vi "Dual output square wave 180 out of phase.vi"(8 "error in (no error)":errorcluster, 11 "VISA resource name":refnum<visa-resource-name>="USB0::0x1AB1::0x0641::DG4E202501630::INSTR") -> (0 "error out":errorcluster)   [LabVIEW 2018]
uses:
  <instrlib>/RIGOL DG4000 Series/Public/Configure/Configure Standard Waveform(Square).vi
  <instrlib>/RIGOL DG4000 Series/Public/Configure/Configure Waveform Characteristics(Shape).vi
  <instrlib>/RIGOL DG4000 Series/Public/Configure/Configure Waveform Characteristics(Phase).vi
  <instrlib>/RIGOL DG4000 Series/RIGOL DG4000 Series.lvlib
panel:
  in  "Duty Cycle (50 %) 1":dbl=45.0
  in  "Duty Cycle (50 %) 2":dbl=45.0
  in  "Phase (0 Degree) 2":dbl
  in  "Phase (0 Degree) 1":dbl
  in  "DC Offset (0 V) 1":dbl=1.65
  in  "DC Offset (0 V) 2":dbl=1.65
  in  "Enable Align (F: Disable) 2":bool=TRUE
  in  "Enable Output 2":bool=TRUE
  in  "Enable Align (F: Disable) 1":bool=TRUE
  in  "Enable Output 1":bool=TRUE
  in  "Frequency 1":dbl
  in  "Frequency 2":dbl=180.0
  in  "Waveform Shape (0: Sinusoid) 2":i32(ring)=1 items=["Sinusoid", "Square", "Ramp", "Pulse", "Noise", "User", "Harmonic", "Custom", "DC", "AbsSine", "AbsSineHalf", "AmpALT", "AttALT", "GaussPulse", "NegRamp", "NPulse", "PPulse", "SineTra", "SineVer", "StairDn", "StairUD", "StairUp", "Trapezia", "BandLimited", "Butterworth", "Chebyshev1", "Chebyshev2", "Combin", "CPulse", "CWPulse", "DampedOsc", "DualTone", "Gamma", "GateVibr", "LEMPulse", "MCNoise", "Discharge", "Pahcur", "Quake", "Radar", "Ripple", "RoundHalf", "RoundPM", "StepResp", "SwingOsc", "TV", "Voice", "AM", "FM", "PM", "PWM", "PFM", "Cardiac", "EOG", "EEG", "EMG", "Pulseilogram", "ResSpeed", "LFPulse", "Tens1", "Tens2", "Tens3", "Lgnition", "ISO16750-2 SP", "ISO16750-2 VR", "ISO7637-2 TP1", "ISO7637-2 TP2A", "ISO7637-2 TP2B", "ISO7637-2 TP3A", "ISO7637-2 TP3B", "ISO7637-2 TP4", "ISO7637-2 TP5A", "ISO7637-2 TP5B", "SCR", "Surge", "Airy", "Besselj", "Bessely", "Cauchy", "Cubic", "Dirichlet", "Erf", "Erfc", "Erfclnv", "Erflnv", "ExpFall", "ExpRise", "Gauss", "HaverSine", "Laguerre", "Laplace", "Legend", "Log", "LogNormal", "Lorentz", "Maxwell", "Rayleigh", "Versiera", "Weibull", "ARB_X2", "CosH", "CosInt", "Cot", "CotHCon", "CotHPro", "CscCon", "CscPro", "CscHCon", "CscHPro", "RecipCon", "RecipPro", "SecCon", "SecPro", "SecH", "Sinc", "SinH", "SinInt", "Sqrt", "Tan", "TanH", "ACos", "ACosH", "ACotCon", "ACotPro", "ACotHCon", "ACotHPro", "ACscCon", "ACscPro", "ACscHCon", "ACscHPro", "ASecCon", "ASsePro", "ASecH", "ASin", "ASinH", "ATan", "ATanH", "Barlett", "BarthannWin", "Blackman", "BlackmanH", "BlackmanWin", "Boxcar", "ChebWin", "FlattopWin", "Hamming", "Hanning", "Kaiser", "NuttallWin", "ParzenWin", "TaylorWin", "Triang", "TukeyWin"]
  in  "Output Channel (1: Channel 1) 2":i32(ring)=2 items=["Channel 1"=1, "Channel 2"=2]
  in  "Amplitude (0.1 Vpp) 2":dbl=3.3
  in  "Amplitude (0.1 Vpp) 1":dbl=3.3
  in  "Output Channel (1: Channel 1)":i32(ring)=1 items=["Channel 1"=1, "Channel 2"=2]
  in  "Waveform Shape (0: Sinusoid) 1":i32(ring)=1 items=["Sinusoid", "Square", "Ramp", "Pulse", "Noise", "User", "Harmonic", "Custom", "DC", "AbsSine", "AbsSineHalf", "AmpALT", "AttALT", "GaussPulse", "NegRamp", "NPulse", "PPulse", "SineTra", "SineVer", "StairDn", "StairUD", "StairUp", "Trapezia", "BandLimited", "Butterworth", "Chebyshev1", "Chebyshev2", "Combin", "CPulse", "CWPulse", "DampedOsc", "DualTone", "Gamma", "GateVibr", "LEMPulse", "MCNoise", "Discharge", "Pahcur", "Quake", "Radar", "Ripple", "RoundHalf", "RoundPM", "StepResp", "SwingOsc", "TV", "Voice", "AM", "FM", "PM", "PWM", "PFM", "Cardiac", "EOG", "EEG", "EMG", "Pulseilogram", "ResSpeed", "LFPulse", "Tens1", "Tens2", "Tens3", "Lgnition", "ISO16750-2 SP", "ISO16750-2 VR", "ISO7637-2 TP1", "ISO7637-2 TP2A", "ISO7637-2 TP2B", "ISO7637-2 TP3A", "ISO7637-2 TP3B", "ISO7637-2 TP4", "ISO7637-2 TP5A", "ISO7637-2 TP5B", "SCR", "Surge", "Airy", "Besselj", "Bessely", "Cauchy", "Cubic", "Dirichlet", "Erf", "Erfc", "Erfclnv", "Erflnv", "ExpFall", "ExpRise", "Gauss", "HaverSine", "Laguerre", "Laplace", "Legend", "Log", "LogNormal", "Lorentz", "Maxwell", "Rayleigh", "Versiera", "Weibull", "ARB_X2", "CosH", "CosInt", "Cot", "CotHCon", "CotHPro", "CscCon", "CscPro", "CscHCon", "CscHPro", "RecipCon", "RecipPro", "SecCon", "SecPro", "SecH", "Sinc", "SinH", "SinInt", "Sqrt", "Tan", "TanH", "ACos", "ACosH", "ACotCon", "ACotPro", "ACotHCon", "ACotHPro", "ACscCon", "ACscPro", "ACscHCon", "ACscHPro", "ASecCon", "ASsePro", "ASecH", "ASin", "ASinH", "ATan", "ATanH", "Barlett", "BarthannWin", "Blackman", "BlackmanH", "BlackmanWin", "Boxcar", "ChebWin", "FlattopWin", "Hamming", "Hanning", "Kaiser", "NuttallWin", "ParzenWin", "TaylorWin", "Triang", "TukeyWin"]
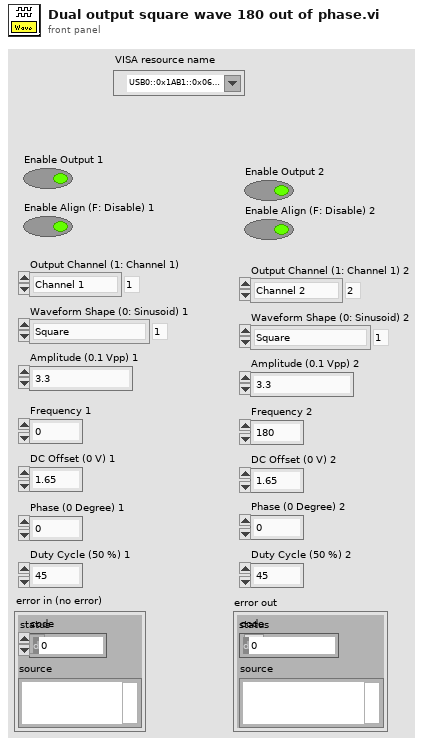
[diagram p1: front panel]
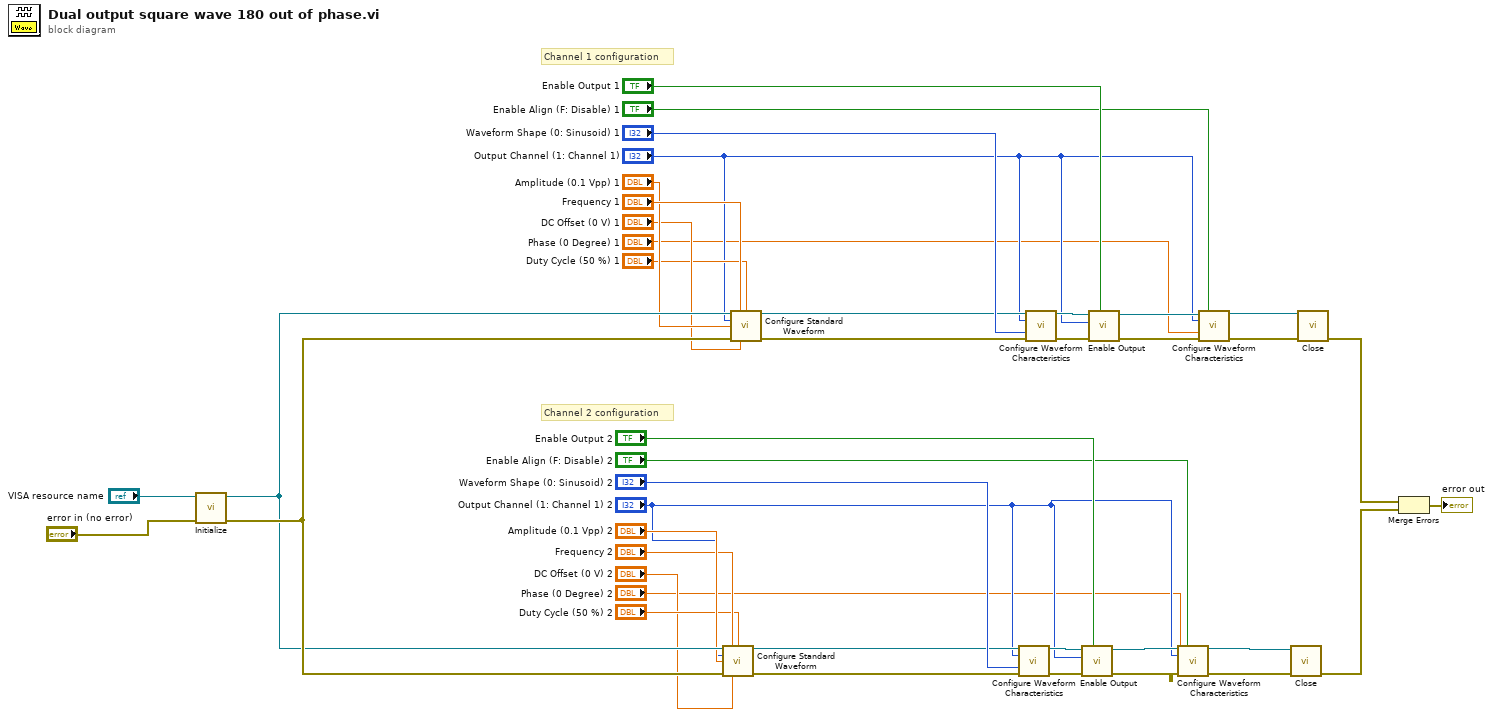
[diagram p0: block diagram]
diagram:
  # "Channel 2 configuration"
  # "Channel 1 configuration"
  n1 = call <instrlib>:"Initialize.vi"("error in (no error)"="error in (no error)", "VISA resource name"="VISA resource name") -> ("error out"=w34:errorcluster, "VISA resource name out"=w31:refnum<visa-resource-name>)  [unwired: 3 in, 5 out]
  n2 = call-poly <instrlib>:"Configure Standard Waveform.vi"("VISA resource name"=w31, "Frequency (1000 Hz)"="Frequency 2", "Output Channel (1: Channel 1)"="Output Channel (1: Channel 1) 2", "Amplitude (5 Vpp)"="Amplitude (0.1 Vpp) 2", "error in (no error)"=w34, "Offset (0)"="DC Offset (0 V) 2", "Duty Cycle (50 %)"="Duty Cycle (50 %) 2") -> ("VISA resource name out"=w26:refnum<visa-resource-name>, "error out"=w25:errorcluster)  [unwired: 7 in]
  n3 = call-poly <instrlib>:"Configure Standard Waveform.vi"("VISA resource name"=w31, "Frequency (1000 Hz)"="Frequency 1", "Output Channel (1: Channel 1)"="Output Channel (1: Channel 1)", "Amplitude (5 Vpp)"="Amplitude (0.1 Vpp) 1", "error in (no error)"=w34, "Offset (0)"="DC Offset (0 V) 1", "Duty Cycle (50 %)"="Duty Cycle (50 %) 1") -> ("VISA resource name out"=w24:refnum<visa-resource-name>, "error out"=w23:errorcluster)  [unwired: 7 in]
  n4 = call-poly <instrlib>:"Configure Waveform Characteristics.vi"("VISA resource name"=w26, "Output Channel (1: Channel 1)"="Output Channel (1: Channel 1) 2", "Waveform Shape (0: Sinusoid)"="Waveform Shape (0: Sinusoid) 2", "error in (no error)"=w25) -> ("VISA resource name out"=w30:refnum<visa-resource-name>, "error out"=w29:errorcluster)  [unwired: 10 out]
  n5 = call-poly <instrlib>:"Configure Waveform Characteristics.vi"("VISA resource name"=w24, "Output Channel (1: Channel 1)"="Output Channel (1: Channel 1)", "Waveform Shape (0: Sinusoid)"="Waveform Shape (0: Sinusoid) 1", "error in (no error)"=w23) -> ("VISA resource name out"=w28:refnum<visa-resource-name>, "error out"=w27:errorcluster)  [unwired: 10 out]
  n6 = call <instrlib>:"Enable Output.vi"("Enable Output (T: Enable)"="Enable Output 2", "error in (no error)"=w29, "Output Channel (1: Channel 1)"="Output Channel (1: Channel 1) 2", "VISA resource name"=w30) -> ("error out"=w8:errorcluster, "VISA resource name out"=w5:refnum<visa-resource-name>)  [unwired: 6 out]
  n7 = call <instrlib>:"Enable Output.vi"("Enable Output (T: Enable)"="Enable Output 1", "error in (no error)"=w27, "Output Channel (1: Channel 1)"="Output Channel (1: Channel 1)", "VISA resource name"=w28) -> ("error out"=w11:errorcluster, "VISA resource name out"=w14:refnum<visa-resource-name>)  [unwired: 6 out]
  n8 = call-poly <instrlib>:"Configure Waveform Characteristics.vi"("VISA resource name"=w5, "Enable Align (F: Disable)"="Enable Align (F: Disable) 2", "Output Channel (1: Channel 1)"="Output Channel (1: Channel 1) 2", "Phase (0 Degree)"="Phase (0 Degree) 2", "error in (no error)"=w8) -> ("VISA resource name out"=w9:refnum<visa-resource-name>, "error out"=w7:errorcluster)  [unwired: 9 in]
  n9 = call-poly <instrlib>:"Configure Waveform Characteristics.vi"("VISA resource name"=w14, "Enable Align (F: Disable)"="Enable Align (F: Disable) 1", "Output Channel (1: Channel 1)"="Output Channel (1: Channel 1)", "Phase (0 Degree)"="Phase (0 Degree) 1", "error in (no error)"=w11) -> ("VISA resource name out"=w13:refnum<visa-resource-name>, "error out"=w12:errorcluster)  [unwired: 9 in]
  n10 = call <instrlib>:"Close.vi"("error in (no error)"=w7, "VISA resource name"=w9) -> ("error out"=w36:errorcluster)  [unwired: 9 out]
  n11 = call <instrlib>:"Close.vi"("error in (no error)"=w12, "VISA resource name"=w13) -> ("error out"=w37:errorcluster)  [unwired: 9 out]
  n12 = Merge Errors(w37, w36) -> (→"error out":errorcluster)
